vi "Fingerprint Length.vi"(8 "Error In":errorcluster, 10 "Type":T1=enum."SHA1", 11 "Session In":refnum<class "Session.lvclass">) -> (0 "Error Out":errorcluster, 2 "Length":i32, 3 "Sesssion Out":refnum<class "Session.lvclass">)   [LabVIEW 2017, in "Toolkit.lvlib" / "Session.lvclass"]
uses:
  Session.lvclass
  Typedefs/Host Key Hash Types.ctl
  Session.lvclass/Session.ctl
  Toolkit.lvlib
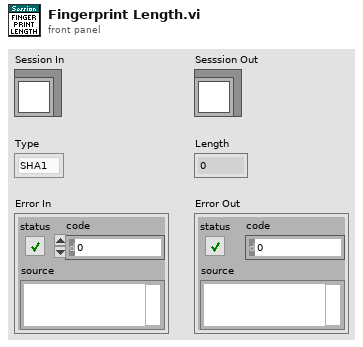
[diagram p1: front panel]
types:
  T1 = typedef "Toolkit.lvlib/Session.lvclass/Host Key Hash Types.ctl" = enum32{"MD5", "SHA1"}
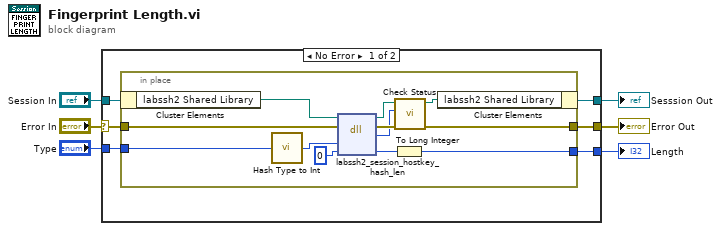
[diagram p0: block diagram]
diagram:
  n1 = case shown="No Error" "Error In" {
    selector: "Error In" -> [w12 w26]
    tunnel: [w8 w26] -> w5
    tunnel: "Session In" -> [w11 w25]
    tunnel: [w10 w25] -> w3
    tunnel: "Type" -> [w9 _]
    tunnel: [w7 _] -> w1
    frame No Error {
      n2 = in-place {
        in-place-border: w12 -> [w20]
        in-place-border: w9 -> [w14]
        in-place-border: [w18] -> w8
        in-place-border: [w15] -> w7
        n3 = in-place-cluster #1(w11) -> ("labssh2 Shared Library"=w24:path)
        n4 = call "Hash Type to Int.vi"("Type"=w14) -> ("i32"=w13:i32)
        n5 = dll-call lib="D:/Users/cfield/Code/Field R&D Services/SSH/LabSSH2/LabVIEW/trunk/src/Toolkit/Support/labssh2.*" fn="labssh2_session_hostkey_hash_len"(path in=w24, error in=w20, "type"=w13, "length"=u64 0) -> (path out=w22:path, error out=w23:errorcluster, "result"=w21:i32, "length"=w16:u64)  [unwired: 2 in]
        n6 = To Long Integer(number=w16) -> (32bit integer=w15:i32)
        n7 = call "Check Status.vi"("Error In"=w23, "Status"=w21, "labssh2 Shared Library In"=w22) -> ("Error Out"=w18:errorcluster, "labssh2 Shared Library Out"=w17:path)  [unwired: 7 in]
        n8 = in-place-cluster #1("labssh2 Shared Library"=w17) -> (w10:refnum<class "Session.lvclass">)
      }
    }
    frame Error {
    }
  }
  "Sesssion Out" <- w3
  "Error Out" <- w5
  "Length" <- w1
